vi "List Linked List Child IDs.vi"(7 "Linked List ID":string, 8 "error in (no error)":errorcluster, 11 "Linked List Ref":refnum<data-value>) -> (0 "error out":errorcluster, 2 "Child IDs":string[](array[string]), 3 "Linked List Ref out":refnum<data-value>)   [LabVIEW 2020, in "Linked Lists.lvlib" / "Linked List Ref.lvclass"]
uses:
  <vilib>/gpm_packages/@cs/linked-list/Source/Linked List/Linked List Ref/Linked List Ref.lvclass
  <vilib>/gpm_packages/@cs/linked-list/Source/Linked List/ILinkedList/ILinked List.lvclass
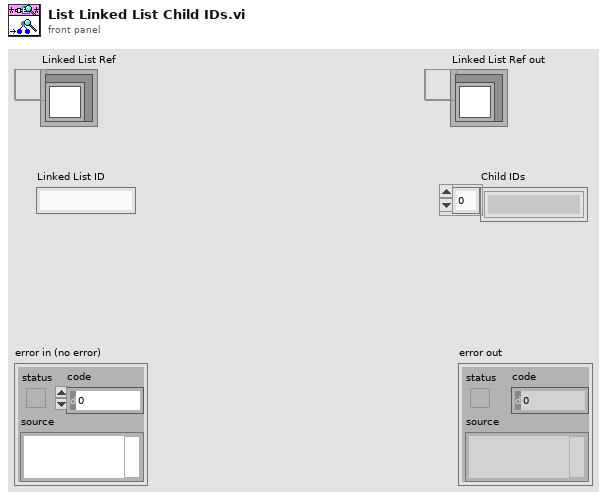
[diagram p1: front panel]
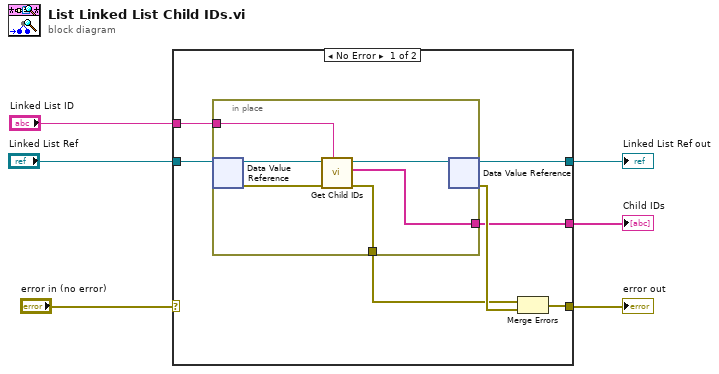
[diagram p0: block diagram]
diagram:
  n1 = case shown="No Error" "error in (no error)" {
    selector: "error in (no error)" -> [_ w20]
    tunnel: "Linked List Ref" -> [w13 w21]
    tunnel: [w12 w21] -> w5
    tunnel: [w11 w20] -> w3
    tunnel: "Linked List ID" -> [w8 _]
    tunnel: [w7 _] -> w1
    frame No Error {
      n2 = in-place {
        in-place-border: [w18] -> w9
        in-place-border: w8 -> [w15]
        in-place-border: [w14] -> w7
        n3 = in-place-dvr #1(w13) -> (w17:refnum<class "ILinked List.lvclass">, w19:errorcluster)
        n4 = call-dynamic "Get Child IDs.vi"("Linked List ID"=w15, "error in (no error)"=w19, "ILinked List in"=w17) -> ("error out"=w18:errorcluster, "Child IDs"=w14:string[], "ILinked List out"=w16:refnum<class "ILinked List.lvclass">)  [unwired: 6 in]
        n5 = in-place-dvr #1(w16) -> (w12:refnum<data-value>, w10:errorcluster)
      }
      n6 = Merge Errors(w9, w10) -> (w11:errorcluster)
    }
    frame Error {
    }
  }
  "error out" <- w3
  "Linked List Ref out" <- w5
  "Child IDs" <- w1
